vi "Write_CmdDiagnostic_Wrapper.vi"(8 "error in (no error)":errorcluster, 10 "Command":T1(ring), 11 "Multiplexer_Opmux in":refnum<class "Multiplexer_Opmux.lvclass">) -> (0 "error out":errorcluster, 3 "Multiplexer_Opmux out":refnum<class "Multiplexer_Opmux.lvclass">)   [LabVIEW 2014, in "Multiplexer_Opmux.lvclass"]
uses:
  Multiplexer_Opmux.lvclass
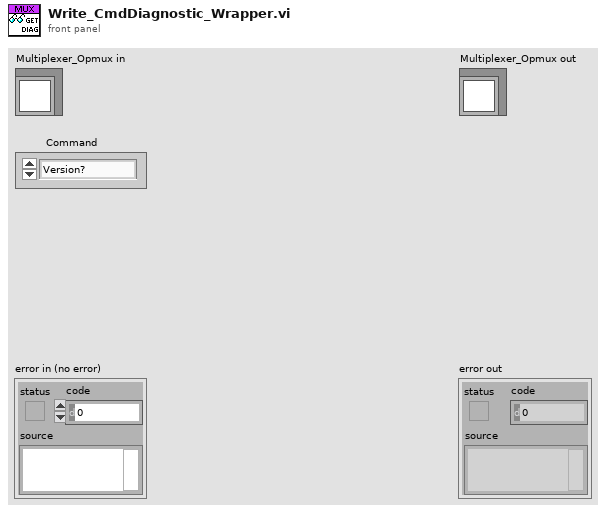
[diagram p1: front panel]
types:
  T1 = enum16{"Version?", "Software Trigger", "Reset", "Radiator Temp?", "In Voltage?"}
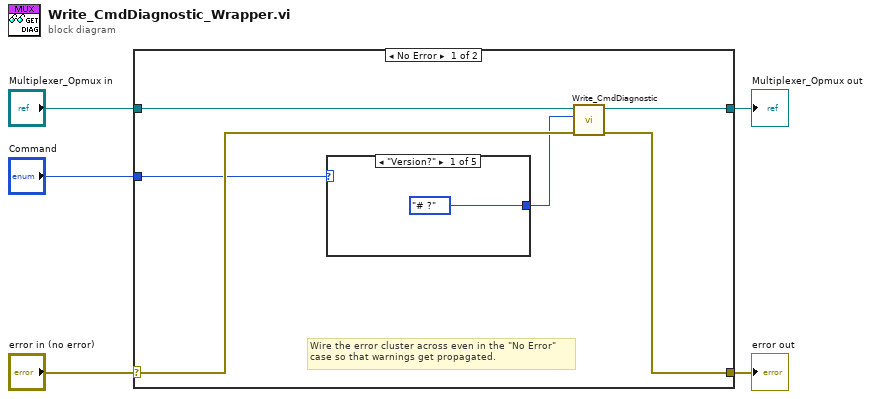
[diagram p0: block diagram]
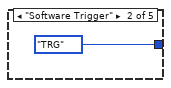
[diagram p2: hidden frame]
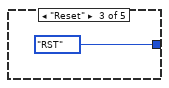
[diagram p3: hidden frame]
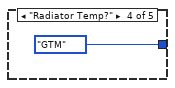
[diagram p4: hidden frame]
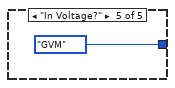
[diagram p5: hidden frame]
diagram:
  n1 = case shown="No Error" "error in (no error)" {
    selector: "error in (no error)" -> [w8 w18]
    tunnel: [w9 w18] -> w4
    tunnel: [w10 w17] -> w2
    tunnel: "Multiplexer_Opmux in" -> [w11 w17]
    tunnel: "Command" -> [w7 _]
    frame No Error {
      # "Wire the error cluster across even in the \"No Error\"\ncase so that warnings get propagated."
      n2 = case shown="\"Version?\"" w7 {
        tunnel: [enum16{"# ?", "TRG", "RST", "GTM", "GVM"}."# ?" ("Command") enum16{"# ?", "TRG", "RST", "GTM", "GVM"}."TRG" ("Command") enum16{"# ?", "TRG", "RST", "GTM", "GVM"}."RST" ("Command") enum16{"# ?", "TRG", "RST", "GTM", "GVM"}."GTM" ("Command") enum16{"# ?", "TRG", "RST", "GTM", "GVM"}."GVM" ("Command")] -> w6
        frame "Version?" {
        }
        frame "Software Trigger" {
        }
        frame "Reset" {
        }
        frame "Radiator Temp?" {
        }
        frame "In Voltage?" {
        }
      }
      n3 = call-dynamic "Write_CmdDiagnostic.vi"("error in (no error)"=w8, "Command"=w6, "Multiplexer_Opmux in"=w11) -> ("error out"=w9:errorcluster, "Multiplexer_Opmux out"=w10:refnum<class "Multiplexer_Opmux.lvclass">)  [unwired: 7 in]
    }
    frame Error {
    }
  }
  "error out" <- w4
  "Multiplexer_Opmux out" <- w2
